vi "lv stream buffer add value.vi"(8 "error in":errorcluster, 9 "data values":dbl[](array[numeric]), 10 "timestamp":i64, 11 "buffer handle":i32) -> (0 "error out":errorcluster, 3 "full":u8)   [LabVIEW 2026]
uses:
  bin/nominalClient_64.dll
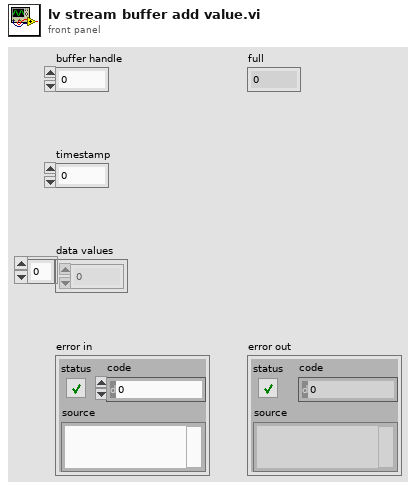
[diagram p1: front panel]
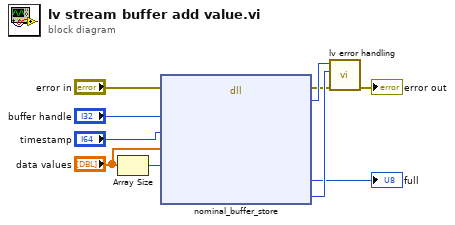
[diagram p0: block diagram]
diagram:
  n1 = Array Size(array="data values") -> (size(s)=w9:i32)
  n2 = dll-call lib="C:/sw/nominal-c/bin/nominalClient_64.dll" fn="nominal_buffer_store"(error in="error in", "buffer"="buffer handle", "timestamp ns"="timestamp", "data values"="data values", "channel count"=w9) -> (error out=w2:errorcluster, "return type"=w5:i32, "full"=→"full":u8, "errorout"=w4:i32)  [unwired: 8 in, 1 out]
  n3 = call "lv error handling.vi"("error in"=w2, "error handle"=w4, "return code"=w5) -> ("error out"=→"error out":errorcluster)  [unwired: 8 in]
